vi "Read_Write_Text_File.vi"(0 "File_Path_In":path, 5 "Data_In":string, 11 "Error_In":errorcluster, 12 "Mode":T1=enum."Read") -> (4 "File_Path_Out":path, 6 "Data_Out":string, 15 "Error_Out":errorcluster)   [LabVIEW 2023, in "File_Handler_Library.lvlib"]
doc: "This VI read or write to the Text file"
uses:
  File_Handler_Library.lvlib
  Library_Controls/Mode.ctl
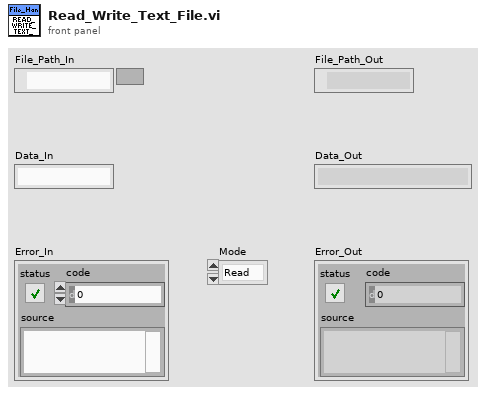
[diagram p1: front panel]
types:
  T1 = typedef "File_Handler_Library.lvlib/Mode.ctl" = enum16{"Write", "Read"}
  T2 = enum16{"open", "replace", "create", "open or create", "replace or create", "replace or create with confirmation"}
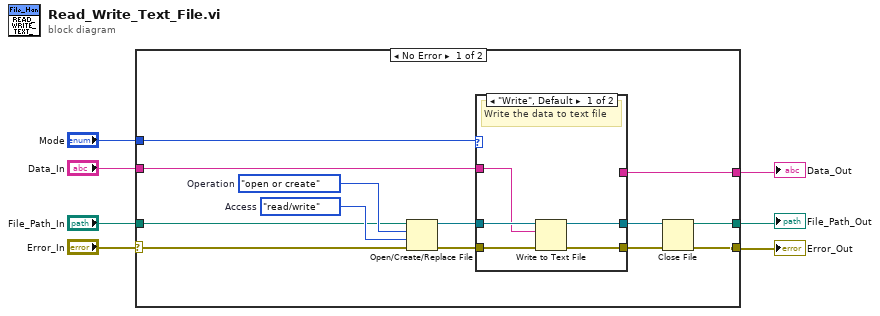
[diagram p0: block diagram]
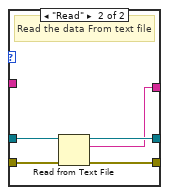
[diagram p2: hidden frame]
diagram:
  n1 = case shown="No Error" "Error_In" {
    selector: "Error_In" -> [w14 w32]
    tunnel: [w13 w32] -> w6
    tunnel: "Mode" -> [w12 _]
    tunnel: "File_Path_In" -> [w11 w31]
    tunnel: "Data_In" -> [w10 _]
    tunnel: [w9 w31] -> w2
    tunnel: [w8 _] -> w1
    frame No Error {
      w17 = enum16{"read/write", "read-only", "write-only"}."read/write"  # Access
      w16 = T2."open or create"  # Operation
      n2 = Open/Create/Replace File(file path (use dialog)=w11, error in=w14, operation (0:open)=w16, access (0:read/write)=w17) -> (refnum out=w18:refnum<file>, error out=w20:errorcluster)  [unwired: 2 in, 1 out]
      n3 = case shown="\"Write\", Default" w12 {
        tunnel: w20 -> [w25 w30]
        tunnel: [w24 w29] -> w19
        tunnel: w18 -> [w23 w27]
        tunnel: w10 -> [w22 _]
        tunnel: [w21 w28] -> w15
        tunnel: [_ w26] -> w8
        frame "Write", Default {
          # "Write the data to text file"
          n4 = Write to Text File(file (use dialog)=w23, text=w22, error in=w25) -> (refnum out=w21:refnum<file>, error out=w24:errorcluster)  [unwired: 1 in, 1 out]
        }
        frame "Read" {
          # "Read the data From text file"
          n5 = Read from Text File(file (use dialog)=w27, error in=w30) -> (refnum out=w28:refnum<file>, text=w26:string, error out=w29:errorcluster)  [unwired: 2 in, 1 out]
        }
      }
      n6 = Close File(refnum=w15, error in=w19) -> (path=w9:path, error out=w13:errorcluster)
    }
    frame Error {
    }
  }
  "Error_Out" <- w6
  "Data_Out" <- w1
  "File_Path_Out" <- w2
